vi "Test1.vi"   [LabVIEW 2020]
uses:
  MelsecMcNet/MelsecMcNet.lvclass
  E:/Git/Libraries/develop/HslCommunication/Abstract PLC Controler/Abs Controler.lvclass
  lModbusRtu/ModbusRtu.lvclass
  InovanceTCP/InovanceModbusTcp.lvclass
  InovanceSerial/InovanceSerialModbusRtu.lvclass
  0d607765-f7c5-42ca-a0c7-c1384099e99d.vi
  92909ad2-5df7-419e-940b-0063d88abf32.vi
  <vilib>/Utility/error.llb/Trim Whitespace.vi
  Abstract PLC Controler/Abs Controler.lvclass
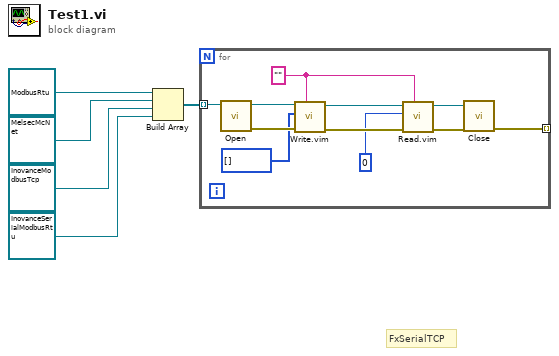
[diagram p0: block diagram]
diagram:
  # "FxSerialTCP"
  n1 = Build Array(refnum<class "ModbusRtu.lvclass"> refnum ("HslCommunication.lvlib:ModbusRtu.lvclass"), refnum<class "MelsecMcNet.lvclass"> refnum ("HslCommunication.lvlib:MelsecMcNet.lvclass"), refnum<class "InovanceModbusTcp.lvclass"> refnum ("HslCommunication.lvlib:InovanceModbusTcp.lvclass"), refnum<class "InovanceSerialModbusRtu.lvclass"> refnum ("HslCommunication.lvlib:InovanceSerialModbusRtu.lvclass")) -> (w4:refnum<class "Abs Controler.lvclass">[])
  n2 = for {
    tunnel: w4 -> [w16] mode=indexing
    tunnel: [w6] -> _ mode=indexing
    w11 = "" ("Start address")
    n3 = call-dynamic "Open.vi"("MelsecTCP in"=w16) -> ("error out"=w14:errorcluster, "MelsecTCP out"=w15:refnum<class "Abs Controler.lvclass">)  [unwired: 9 in]
    n4 = call "Write.vim"("Start address"=w11, "error in (no error)"=w14, "Data"=u64[] [], "MelsecTCP in"=w15) -> ("error out"=w8:errorcluster, "MelsecTCP out"=w9:refnum<class "Abs Controler.lvclass">)  [unwired: 6 in]
    n5 = call "Read.vim"("Start address"=w11, "error in (no error)"=w8, "Read Type"=u64 0 ("Data"), "MelsecTCP in"=w9) -> ("error out"=w12:errorcluster, "MelsecTCP out"=w13:refnum<class "Abs Controler.lvclass">)  [unwired: 5 in, 1 out]
    n6 = call-dynamic "Close.vi"("error in (no error)"=w12, "MelsecTCP in"=w13) -> ("error out"=w6:errorcluster)  [unwired: 8 in, 1 out]
  }
